vi "Read Pixels and Copy to Display Image.vi"(0 "fpga interface in":refnum<k20>, 1 "Ctl Refnum":refnum<vi>, 5 "display channel number":i32, 7 "serial channel display parameters":T4[](array[typedef]) {"RAW parameters"."bayer parameters"."blue gain" format="%_4g"; "RAW parameters"."bayer parameters"."green gain" format="%_4g"; "RAW parameters"."bayer parameters"."red gain" format="%_4g"; "RAW parameters"."bayer parameters"."algorithm" items=["Bilinear", "VNG"]; "RAW parameters"."bayer parameters"."pattern" items=["GB", "GR", "BG", "RG"]}, 9 "image metadata":T2, 11 "error in (no error)":errorcluster) -> (4 "fpga interface out":refnum<k20>, 6 "display image":T1, 15 "error out":errorcluster)   [LabVIEW 2025, in "GettingStarted_Common_148X_Host.lvlib"]
uses:
  GettingStarted_Common_148X_Host.lvlib
  Types/Serial Channel Display Parameters.ctl
  <vilib>/vision/Image Controls.llb/IMAQ Image.ctl
  Types/RAW Interpretation for Display.ctl
  FPGA/Common/Types/Image Metadata.ctl
  <instrlib>/FlexRIO/CSI-2/v2/Common/Types/LLP Data Type.ctl
  <instrlib>/FlexRIO/CSI-2/v2/Common/NI CSI-2 API Common v2.lvlib
  FPGA/Common/GettingStarted_Common_148X_FPGA.lvlib
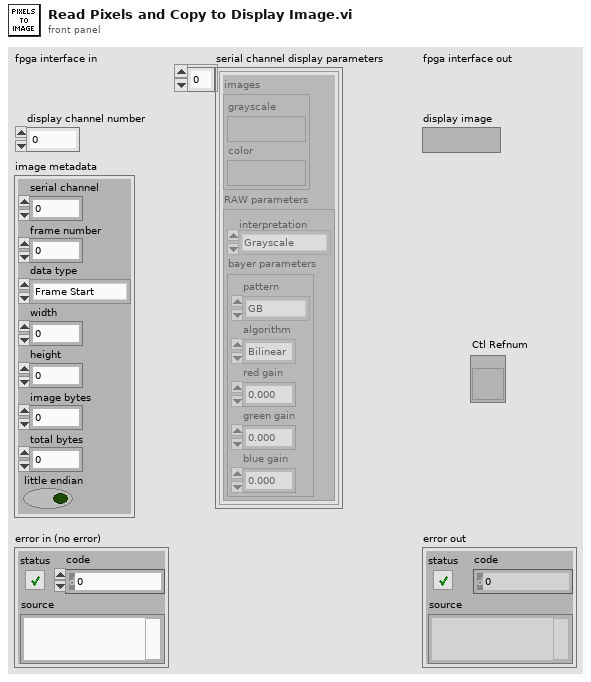
[diagram p1: front panel]
types:
  T1 = typedef "IMAQ Image.ctl" = refnum<image>
  T2 = typedef "GettingStarted_Common_148X_FPGA.lvlib/Image Metadata.ctl" = cluster{"serial channel":fxp<+,3,3>, "frame number":u16, "data type":T3, "width":u16, "height":u16, "image bytes":u32, "total bytes":u32, "little endian":bool}
  T3 = typedef "NI CSI-2 API Common v2.lvlib/LLP Data Type.ctl" = enum8{"Frame Start", "Frame End", "Line Start", "Line End", "End of Transmission", "Reserved 0", "Reserved 1", "Reserved 2", "Generic Short Packet 1", "Generic Short Packet 2", "Generic Short Packet 3", "Generic Short Packet 4", "Generic Short Packet 5", "Generic Short Packet 6", "Generic Short Packet 7", "Generic Short Packet 8", "Null", "Blanking Data", "Embedded 8-bit non Image Data", "Generic Long Packet 1", "Generic Long Packet 2", "Generic Long Packet 3", "Generic Long Packet 4", "Reserved 3", "YUV420 8-bit", "YUV420 10-bit", "Legacy YUV420 8-bit", "Reserved 4", "YUV420 8-bit Chroma Shifted", "YUV420 10-bit Chroma Shifted", "YUV422 8-bit", "YUV422 10-bit", "RGB444", "RGB555", "RGB565", "RGB666", "RGB888", "Reserved 5", "Reserved 6", "RAW 24", "RAW 6", "RAW 7", "RAW 8", "RAW 10", "RAW 12", "RAW 14", "RAW 16", "RAW 20", "User Defined 8-bit Data 1", "User Defined 8-bit Data 2", "User Defined 8-bit Data 3", "User Defined 8-bit Data 4", "User Defined 8-bit Data 5", "User Defined 8-bit Data 6", "User Defined 8-bit Data 7", "User Defined 8-bit Data 8", "USL Command", "Reserved 7", "Reserved 8", "Reserved 9", "Reserved 10", "Reserved 11", "Reserved 12", "LRTE EPD Spacer"}
  T4 = typedef "GettingStarted_Common_148X_Host.lvlib/Serial Channel Display Parameters.ctl" = cluster{"images":cluster{"grayscale":T1, "color":T1}, "RAW parameters":cluster{"interpretation":T5, "bayer parameters":cluster{"pattern":i32, "algorithm":i32, "red gain":dbl, "green gain":dbl, "blue gain":dbl}}}
  T5 = typedef "GettingStarted_Common_148X_Host.lvlib/RAW Interpretation for Display.ctl" = enum16{"Grayscale", "Bayer", "RGB", "YUV422", "YUV420", "Legacy YUV420"}
  T6 = cluster{"pattern":i32, "algorithm":i32, "red gain":dbl, "green gain":dbl, "blue gain":dbl}
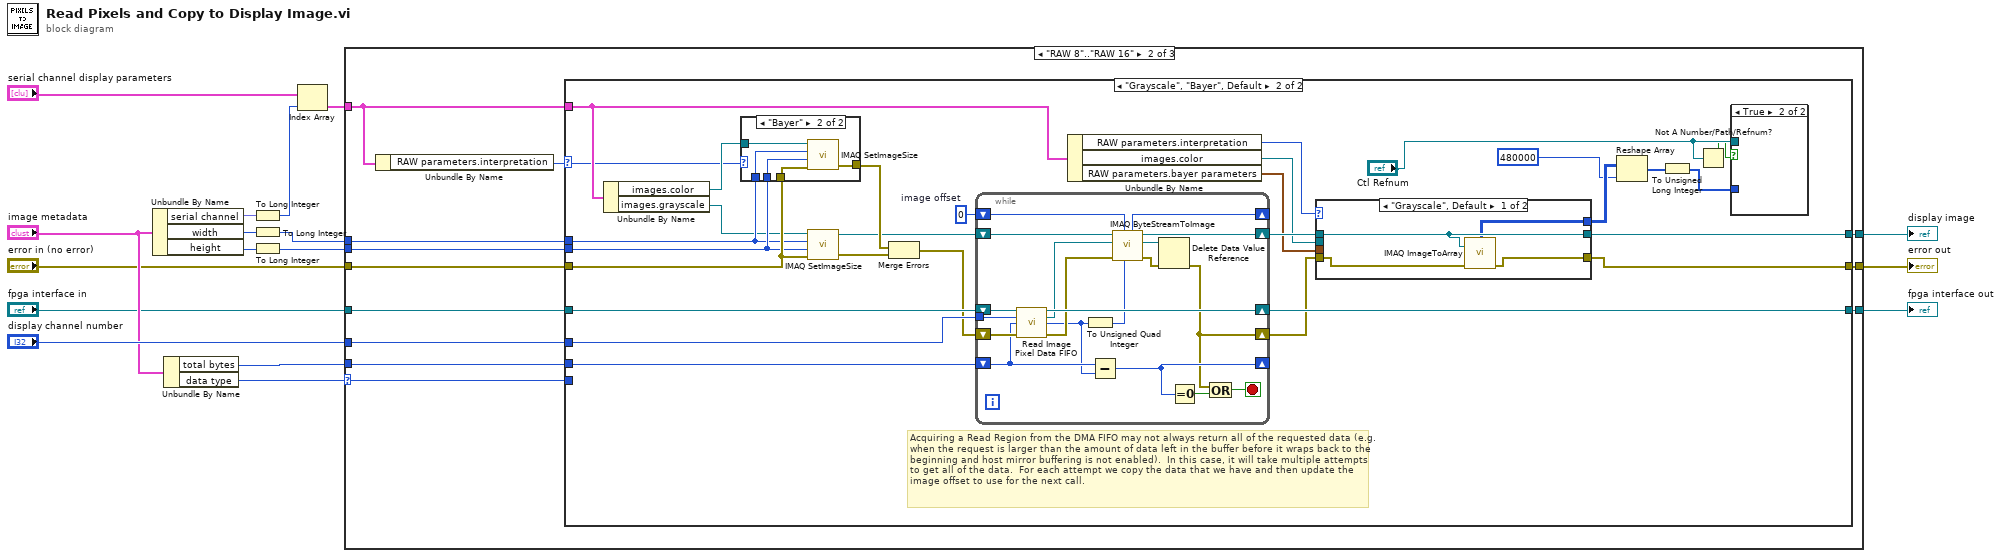
[diagram p0: block diagram]
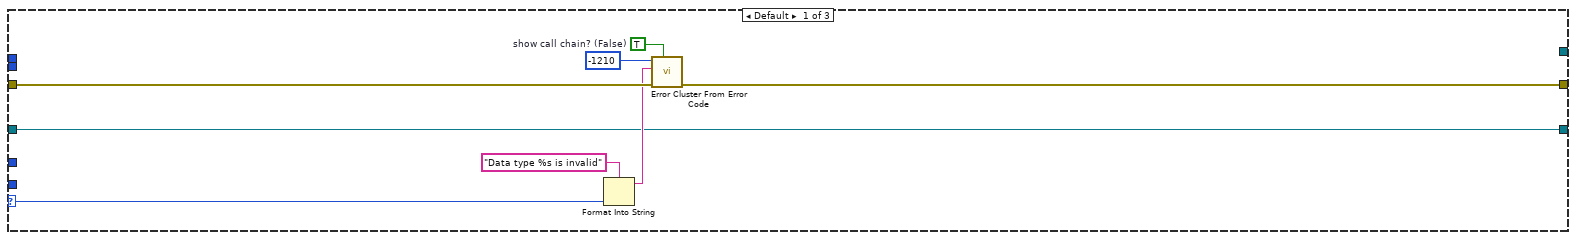
[diagram p2: hidden frame]
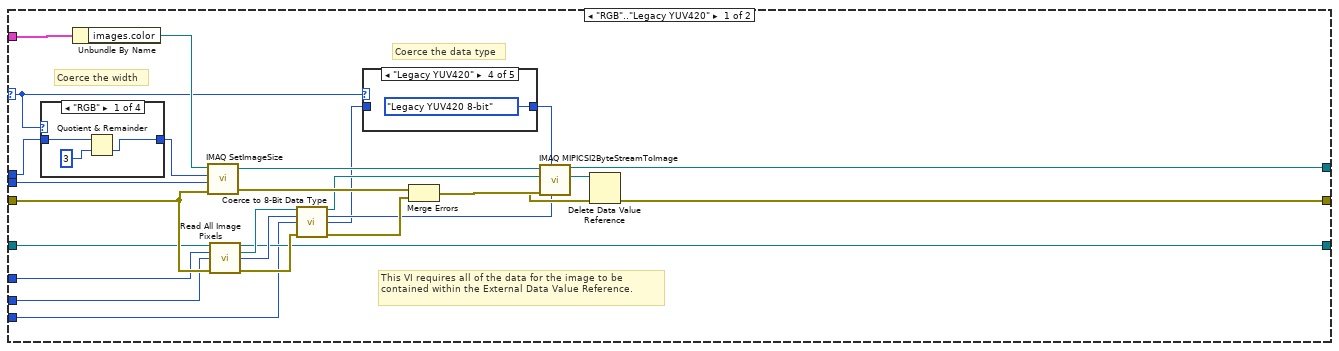
[diagram p3: hidden frame]
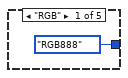
[diagram p4: hidden frame]
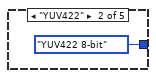
[diagram p5: hidden frame]
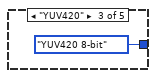
[diagram p6: hidden frame]
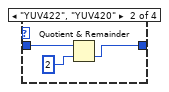
[diagram p8: hidden frame]
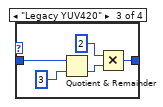
[diagram p9: hidden frame]
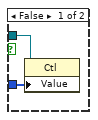
[diagram p11: hidden frame]
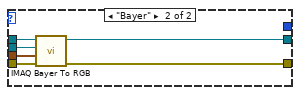
[diagram p13: hidden frame]
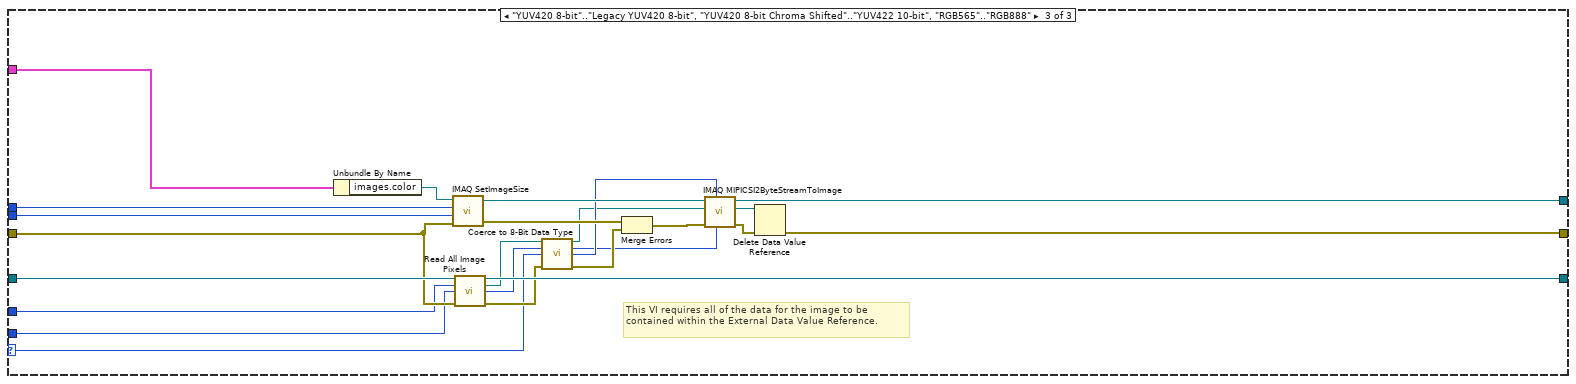
[diagram p14: hidden frame]
diagram:
  n1 = Unbundle By Name("image metadata") -> ("serial channel"=w13:fxp<+,3,3>, "width"=w9:u16, "height"=w10:u16)
  n2 = Unbundle By Name("image metadata") -> ("total bytes"=w16:u32, "data type"=w1:T3)
  n3 = To Long Integer(number=w13) -> (32bit integer=w11:i32)
  n4 = To Long Integer(number=w9) -> (32bit integer=w6:i32)
  n5 = To Long Integer(number=w10) -> (32bit integer=w7:i32)
  n6 = Index Array(array="serial channel display parameters", index=w11) -> (element=w3:T4)
  n7 = case shown="\"RAW 8\"..\"RAW 16\"" w1 {
    selector: w1 -> [w19 w26 w151]
    tunnel: w16 -> [_ w37 w161]
    tunnel: [w18 w36 w163] -> w15
    tunnel: "display channel number" -> [_ w35 w160]
    tunnel: "error in (no error)" -> [w23 w34 w164]
    tunnel: w7 -> [_ w33 w171]
    tunnel: w6 -> [_ w32 w170]
    tunnel: [_ w31 w159] -> w5
    tunnel: [w22 w30 w156] -> w4
    tunnel: w3 -> [_ w28 w168]
    tunnel: "fpga interface in" -> [w18 w29 w167]
    frame Default {
      w24 = TRUE  # show call chain? (False)
      n8 = Format Into String(format string="Data type %s is invalid" ("error message (\"\")"), w19) -> (resulting string=w20:string)  [unwired: 2 in, 1 out]
      n9 = call <vilib>:"Error Cluster From Error Code.vi"("show call chain? (False)"=w24, "error in (no error)"=w23, "error message (\"\")"=w20, "error code (0)"=-1210) -> ("error out"=w22:errorcluster)  [unwired: 5 in]
    }
    frame "RAW 8".."RAW 16" {
      n10 = Unbundle By Name(w28) -> ("RAW parameters.interpretation"=w27:T5)
      n11 = case shown="\"Grayscale\", \"Bayer\", Default" w27 {
        selector: w27 -> [w40 w88]
        tunnel: w37 -> [w47 w110]
        tunnel: [w51 w108] -> w36
        tunnel: w35 -> [w46 w107]
        tunnel: w34 -> [w52 w106]
        tunnel: w33 -> [w43 w104]
        tunnel: w32 -> [w42 w103]
        tunnel: [w49 w100] -> w31
        tunnel: [w50 w98] -> w30
        tunnel: w28 -> [w45 w93]
        tunnel: w29 -> [w48 w92]
        tunnel: w26 -> [w44 _]
        frame "RGB".."Legacy YUV420" {
          # "Coerce the data type"
          # "Coerce the width"
          # "This VI requires all of the data for the image to be contained within the External Data Value Reference."
          n12 = case shown="\"RGB\"" w40 {
            tunnel: w42 -> [w71 w74 w80 w81]
            tunnel: [w70 w73 w77 w81] -> w41
            frame "RGB" {
              n13 = Quotient & Remainder(x=w71, y=3) -> (floor(x/y)=w70:i32)  [unwired: 1 out]
            }
            frame "YUV422", "YUV420" {
              n14 = Quotient & Remainder(x=w74, y=2) -> (floor(x/y)=w73:i32)  [unwired: 1 out]
            }
            frame "Legacy YUV420" {
              n15 = Quotient & Remainder(x=w80, y=3) -> (floor(x/y)=w78:i32)  [unwired: 1 out]
              n16 = Multiply(x=2, y=w78) -> (x*y=w77:i32)
            }
            frame Default {
            }
          }
          n17 = Unbundle By Name(w45) -> ("images.color"=w64:T1)
          n18 = call "IMAQ SetImageSize"("error in (no error)"=w52, "Y Resolution"=w43, "X Resolution"=w41, "Image"=w64) -> ("error out"=w62:errorcluster, "Image Out"=w63:T1)  [unwired: 1 in]
          n19 = call "Read All Image Pixels.vi"("fpga inteface in"=w48, "display channel number"=w46, "image bytes"=w47, "error in (no error)"=w52) -> ("fpga interface out"=w51:refnum<k20>, "image pixel data region"=w57:refnum<data-value>, "elements in region"=w56:u32, "error out"=w58:errorcluster)  [unwired: 8 in]
          n20 = call "Coerce to 8-Bit Data Type.vi"("image pixel data region in"=w57, "image bytes in"=w56, "data type in"=w44, "error in (no error)"=w58) -> ("image pixel data region out"=w53:refnum<data-value>, "image bytes out"=w54:u32, "data type out"=w38:T3, "error out"=w55:errorcluster)  [unwired: 8 in]
          n21 = case shown="\"Legacy YUV420\"" w40 {
            tunnel: w38 -> [_ _ _ _ w69]
            tunnel: [LLP_Data_Type."RGB888" ("data type") LLP_Data_Type."YUV422 8-bit" ("data type") LLP_Data_Type."YUV420 8-bit" ("data type") LLP_Data_Type."Legacy YUV420 8-bit" ("data type") w69] -> w39
            frame "RGB" {
            }
            frame "YUV422" {
            }
            frame "YUV420" {
            }
            frame "Legacy YUV420" {
            }
            frame Default {
            }
          }
          n22 = Merge Errors(w62, w55) -> (w61:errorcluster)
          n23 = call "IMAQ MIPICSI2ByteStreamToImage"("Bytes to Copy"=w54, "Format"=w39, "error in (no error)"=w61, "Byte Stream In"=w53, "Image In"=w63) -> ("error out"=w60:errorcluster, "Byte Stream Out"=w59:refnum<data-value>, "Image Out"=w49:T1)  [unwired: 3 in, 1 out]
          n24 = Delete Data Value Reference(data value reference=w59, error in=w60) -> (error out=w50:errorcluster)  [unwired: 1 out]
        }
        frame "Grayscale", "Bayer", Default {
          w89 = u32 0  # image offset
          # "Acquiring a Read Region from the DMA FIFO may not always return all of the requested data (e.g. when the request is larger than the amount of data left in the buffer before it wraps back to the beginning and host mirror buffering is not enabled).  In this case, it will take multiple attempts to get all of the data.  For each attempt we copy the data that we have and then update the image offset to use for the next call."
          n25 = Unbundle By Name(w93) -> ("images.color"=w102:T1, "images.grayscale"=w97:T1)
          n26 = case shown="\"Bayer\"" w88 {
            tunnel: w106 -> [w113 w118]
            tunnel: [w113 w117] -> w105
            tunnel: w102 -> [_ w116]
            tunnel: w104 -> [_ w115]
            tunnel: w103 -> [_ w114]
            frame "Grayscale", Default {
            }
            frame "Bayer" {
              n27 = call "IMAQ SetImageSize"("error in (no error)"=w118, "Y Resolution"=w115, "X Resolution"=w114, "Image"=w116) -> ("error out"=w117:errorcluster)  [unwired: 1 in, 1 out]
            }
          }
          n28 = call "IMAQ SetImageSize"("error in (no error)"=w106, "Y Resolution"=w104, "X Resolution"=w103, "Image"=w97) -> ("error out"=w109:errorcluster, "Image Out"=w91:T1)  [unwired: 1 in]
          n29 = Merge Errors(w105, w109) -> (w90:errorcluster)
          n30 = while {
            tunnel: w107 -> [w135]
            shift-right: [w136] -> w108
            shift-left: w92 -> [w137]
            shift-right: [w121] -> w99
            shift-left: w90 -> [w134]
            shift-right: [w132] -> w101
            shift-left: w91 -> [w133]
            shift-right: [w124] -> _
            shift-left: w110 -> [w126]
            shift-right: [w120] -> _
            shift-left: w89 -> [w119]
            stop <- w122 stop-if-true
            n31 = call "Read Image Pixel Data FIFO.vi"("fpga inteface in"=w137, "display channel number"=w135, "number of elements"=w126, "error in (no error)"=w134) -> ("fpga interface out"=w136:refnum<k20>, "image pixel data region"=w131:refnum<data-value>, "elements in region"=w125:u32, "error out"=w130:errorcluster)  [unwired: 7 in, 1 out]
            n32 = To Unsigned Quad Integer(1:w125) -> (0:w129:u64)
            n33 = Subtract(x=w126, y=w125) -> (x-y=w124:u32)
            n34 = call "IMAQ ByteStreamToImage"("Bytes to Copy"=w129, "Image Byte Offset In"=w119, "error in (no error)"=w130, "Byte Stream In"=w131, "Image In"=w133) -> ("error out"=w127:errorcluster, "Byte Stream Out"=w128:refnum<data-value>, "Image Out"=w132:T1, "Image Byte Offset Out"=w120:u32)  [unwired: 2 in, 1 out]
            n35 = Delete Data Value Reference(data value reference=w128, error in=w127) -> (error out=w121:errorcluster)  [unwired: 1 out]
            n36 = Equal To 0?(x=w124) -> (x = 0?=w123:bool)
            n37 = Compound Arithmetic op=OR(w121, w123) -> (w122:bool)
          }
          n38 = Unbundle By Name(w93) -> ("RAW parameters.interpretation"=w94:T5, "images.color"=w95:T1, "RAW parameters.bayer parameters"=w96:T6)
          n39 = case shown="\"Grayscale\", Default" w94 {
            tunnel: w101 -> [w139 w147]
            tunnel: [w139 w146] -> w100
            tunnel: w99 -> [w141 w145]
            tunnel: [w140 w144] -> w98
            tunnel: w95 -> [_ w143]
            tunnel: w96 -> [_ w142]
            tunnel: [w138 _] -> w87
            frame "Grayscale", Default {
              n40 = call "IMAQ ImageToArray"("error in (no error)"=w141, "Image"=w139) -> ("error out"=w140:errorcluster, "Image Pixels (U8)"=w138:u8[][])  [unwired: 2 in, 3 out]
            }
            frame "Bayer" {
              n41 = call "IMAQ Bayer To RGB"("error in (no error)"=w145, "Bayer Parameters"=w142, "Image Dst"=w143, "Image Src"=w147) -> ("error out"=w144:errorcluster, "Image Dst Out"=w146:T1)  [unwired: 6 in]
            }
          }
          n42 = Reshape Array(w87, 480000 ("dimension size")) -> (w86:u8[])
          n43 = To Unsigned Long Integer(number=w86) -> (unsigned 32bit integer=w85:u32[])
          n44 = Not A Number/Path/Refnum?(number/path/refnum="Ctl Refnum") -> (NaN/Path/Refnum?=w82:bool)
          n45 = case shown="True" w82 {
            tunnel: w85 -> [w112 _]
            tunnel: "Ctl Refnum" -> [w111 _]
            frame False {
              n46 = property class="Ctl"(reference=w111, "Value"=w112) -> ()  [unwired: 1 in, 2 out]
            }
            frame True {
            }
          }
        }
      }
    }
    frame "YUV420 8-bit".."Legacy YUV420 8-bit", "YUV420 8-bit Chroma Shifted".."YUV422 10-bit", "RGB565".."RGB888" {
      # "This VI requires all of the data for the image to be contained within the External Data Value Reference."
      n47 = Unbundle By Name(w168) -> ("images.color"=w169:T1)
      n48 = call "IMAQ SetImageSize"("error in (no error)"=w164, "Y Resolution"=w171, "X Resolution"=w170, "Image"=w169) -> ("error out"=w165:errorcluster, "Image Out"=w166:T1)  [unwired: 1 in]
      n49 = call "Read All Image Pixels.vi"("fpga inteface in"=w167, "display channel number"=w160, "image bytes"=w161, "error in (no error)"=w164) -> ("fpga interface out"=w163:refnum<k20>, "image pixel data region"=w154:refnum<data-value>, "elements in region"=w153:u32, "error out"=w155:errorcluster)  [unwired: 8 in]
      n50 = call "Coerce to 8-Bit Data Type.vi"("image pixel data region in"=w154, "image bytes in"=w153, "data type in"=w151, "error in (no error)"=w155) -> ("image pixel data region out"=w148:refnum<data-value>, "image bytes out"=w149:u32, "data type out"=w150:T3, "error out"=w152:errorcluster)  [unwired: 8 in]
      n51 = Merge Errors(w165, w152) -> (w162:errorcluster)
      n52 = call "IMAQ MIPICSI2ByteStreamToImage"("Bytes to Copy"=w149, "Format"=w150, "error in (no error)"=w162, "Byte Stream In"=w148, "Image In"=w166) -> ("error out"=w158:errorcluster, "Byte Stream Out"=w157:refnum<data-value>, "Image Out"=w159:T1)  [unwired: 3 in, 1 out]
      n53 = Delete Data Value Reference(data value reference=w157, error in=w158) -> (error out=w156:errorcluster)  [unwired: 1 out]
    }
  }
  "display image" <- w5
  "fpga interface out" <- w15
  "error out" <- w4
